vi "CRYSet Auto Save Front Panel.vi"(11 "Vi Ref":refnum<vi>) -> ()   [LabVIEW 2013]
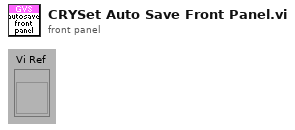
[diagram p1: front panel]
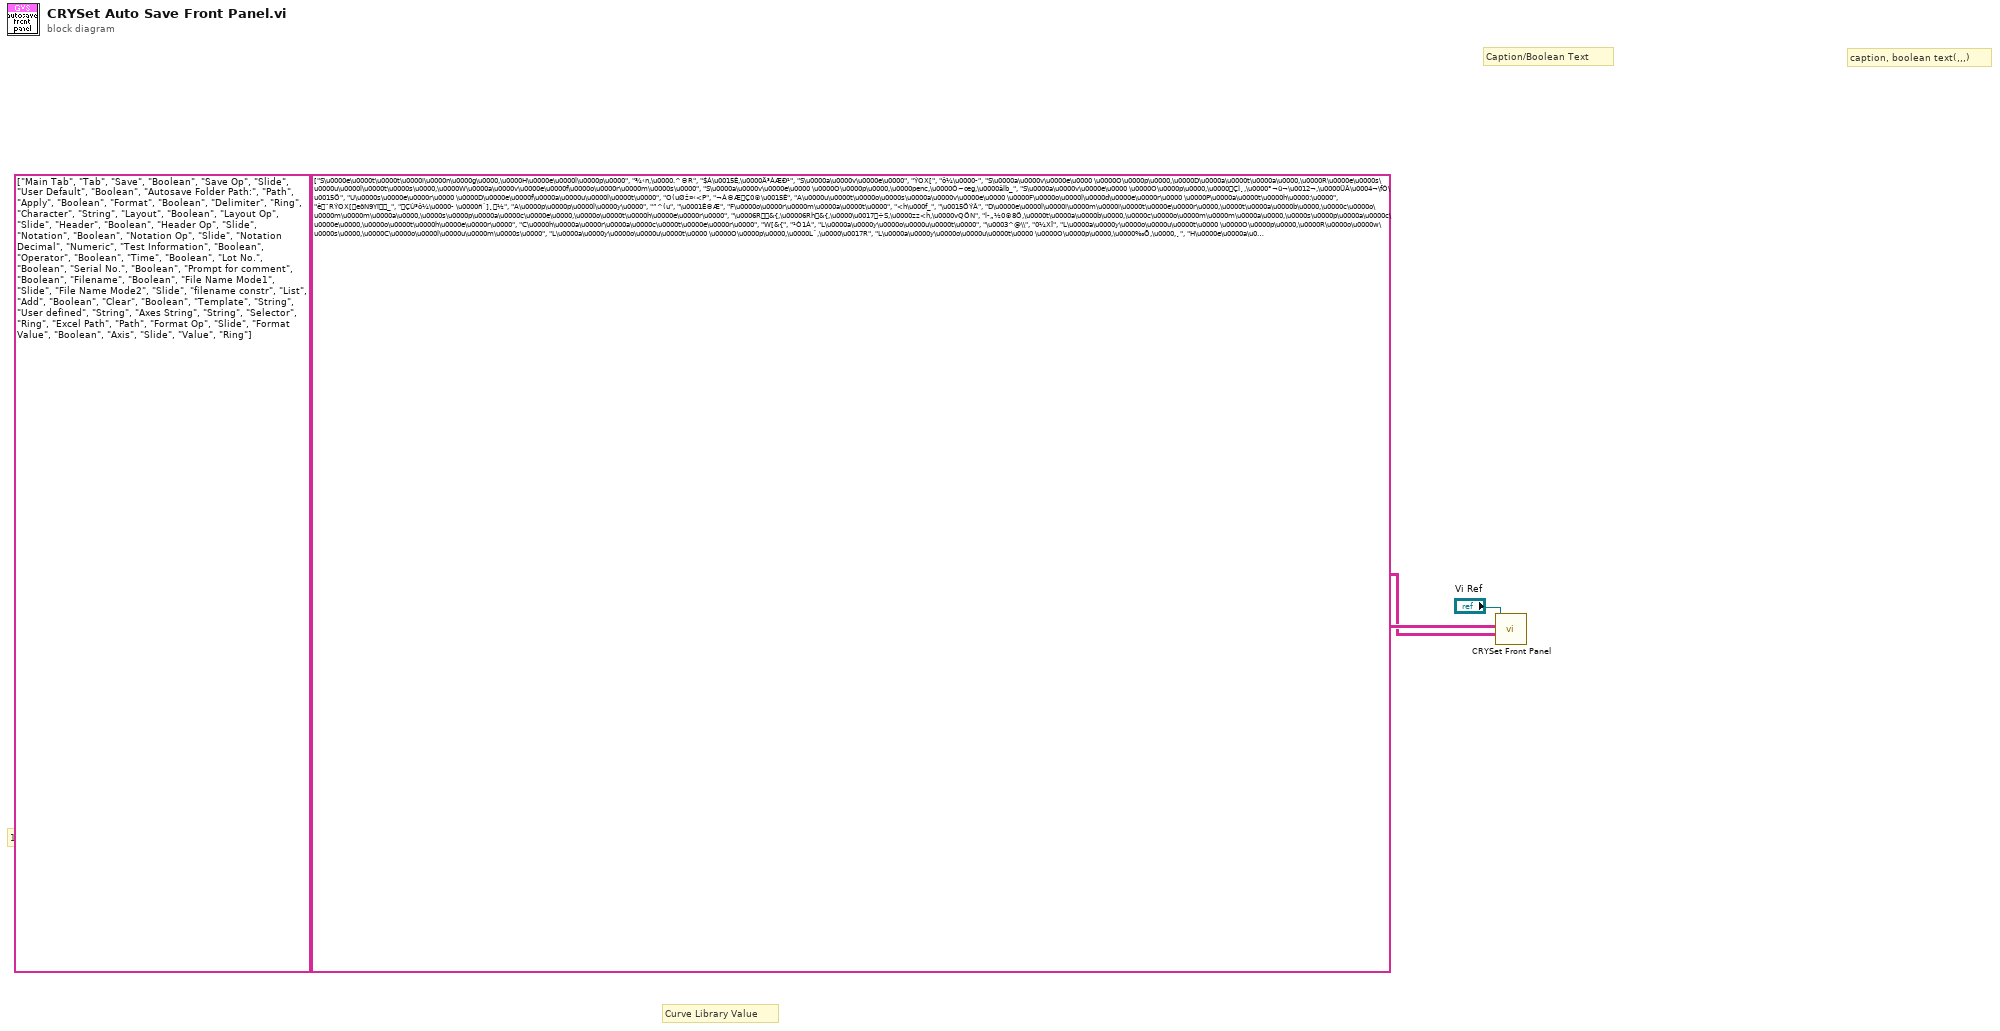
[diagram p0: block diagram]
diagram:
  # "1111"
  # "Curve Library Value"
  # "Caption, Tab Page, Multilist Header, Button 4"
  # "Control Type"
  # "Control Name and Tab"
  # "caption, boolean text(,,,)"
  # "Caption/Boolean Text"
  n1 = call "CRYSet Front Panel.vi"("Caption(Boolean Text)"=string[][] [["S\u0000e\u0000t\u0000t\u0000i\u0000n\u0000g\u0000,\u0000H\u0000e\u0000l\u0000p\u0000", "¾‹n,\u0000.^©R", "$Á\u0015È,\u0000Ä³ÀÆÐ¹"], ["S\u0000a\u0000v\u0000e\u0000", "ÝOX[", "ô¼\u0000­"], ["S\u0000a\u0000v\u0000e\u0000 \u0000O\u0000p\u0000,\u0000D\u0000a\u0000t\u0000a\u0000,\u0000R\u0000e\u0000s\u0000u\u0000l\u0000t\u0000s\u0000,\u0000W\u0000a\u0000v\u0000e\u0000f\u0000o\u0000r\u0000m\u0000s\u0000", "S\u0000a\u0000v\u0000e\u0000 \u0000O\u0000p\u0000,\u0000penc,\u0000Ó~œg,\u0000âlb_", "S\u0000a\u0000v\u0000e\u0000 \u0000O\u0000p\u0000,\u0000ÇÌ¸,\u0000°¬ü¬\u0012¬,\u0000ÜÂ\u0004¬\fÓ\u0015Ö"], ["U\u0000s\u0000e\u0000r\u0000 \u0000D\u0000e\u0000f\u0000a\u0000u\u0000l\u0000t\u0000", "O(uØž¤‹<P", "¬À©ÆÇ0®\u0015È"], ["A\u0000u\u0000t\u0000o\u0000s\u0000a\u0000v\u0000e\u0000 \u0000F\u0000o\u0000l\u0000d\u0000e\u0000r\u0000 \u0000P\u0000a\u0000t\u0000h\u0000:\u0000", "ê¨RÝOX[eöN9Yï_", "ÇÙ³ô¼\u0000­ \u0000ñ´]¸½"], ["A\u0000p\u0000p\u0000l\u0000y\u0000", "”^(u", "\u0001È©Æ"], ["F\u0000o\u0000r\u0000m\u0000a\u0000t\u0000", "<h\u000f_", "\u0015ÖÝÂ"], ["D\u0000e\u0000l\u0000i\u0000m\u0000i\u0000t\u0000e\u0000r\u0000,\u0000t\u0000a\u0000b\u0000,\u0000c\u0000o\u0000m\u0000m\u0000a\u0000,\u0000s\u0000p\u0000a\u0000c\u0000e\u0000,\u0000o\u0000t\u0000h\u0000e\u0000r\u0000", "\u0006R&{,\u00006Rh&{,\u0000\u0017÷S,\u0000zz<h,\u0000vQÖN", "l­„½0®8Ö,\u0000t\u0000a\u0000b\u0000,\u0000c\u0000o\u0000m\u0000m\u0000a\u0000,\u0000s\u0000p\u0000a\u0000c\u0000e\u0000,\u0000o\u0000t\u0000h\u0000e\u0000r\u0000"], ["C\u0000h\u0000a\u0000r\u0000a\u0000c\u0000t\u0000e\u0000r\u0000", "W[&{", "¹Ò1Á"], ["L\u0000a\u0000y\u0000o\u0000u\u0000t\u0000", "\u0003^@\\", "0¼XÎ"], ["L\u0000a\u0000y\u0000o\u0000u\u0000t\u0000 \u0000O\u0000p\u0000,\u0000R\u0000o\u0000w\u0000s\u0000,\u0000C\u0000o\u0000l\u0000u\u0000m\u0000s\u0000", "L\u0000a\u0000y\u0000o\u0000u\u0000t\u0000 \u0000O\u0000p\u0000,\u0000Lˆ,\u0000\u0017R", "L\u0000a\u0000y\u0000o\u0000u\u0000t\u0000 \u0000O\u0000p\u0000,\u0000‰Õ,\u0000,¸"], ["H\u0000e\u0000a\u0000d\u0000e\u0000r\u0000", "\u0007h˜˜", "8º¬¹€½"], ["H\u0000e\u0000a\u0000d\u0000e\u0000r\u0000 \u0000O\u0000p\u0000,\u0000N\u0000o\u0000n\u0000e\u0000,\u0000S\u0000t\u0000a\u0000n\u0000d\u0000a\u0000r\u0000d\u0000,\u0000C\u0000u\u0000s\u0000t\u0000o\u0000m\u0000", "H\u0000e\u0000a\u0000d\u0000e\u0000r\u0000 \u0000O\u0000p\u0000,\u0000àe,\u0000\u0007hÆQ,\u0000ê[IN", "H\u0000e\u0000a\u0000d\u0000e\u0000r\u0000 \u0000O\u0000p\u0000,\u0000ÆÅLÇ,\u0000\\Ô\u0000É,\u0000Ç´Ì\u0015ÈXÇ"], ["N\u0000o\u0000t\u0000a\u0000t\u0000i\u0000o\u0000n\u0000", "&{÷S", "€½8Ö"], ["N\u0000o\u0000t\u0000a\u0000t\u0000i\u0000o\u0000n\u0000 \u0000O\u0000p\u0000,\u0000S\u0000c\u0000i\u0000e\u0000n\u0000t\u0000i\u0000f\u0000i\u0000c\u0000,\u0000F\u0000l\u0000o\u0000a\u0000t\u0000i\u0000n\u0000g\u0000 \u0000p\u0000o\u0000i\u0000n\u0000t\u0000", "N\u0000o\u0000t\u0000a\u0000t\u0000i\u0000o\u0000n\u0000 \u0000O\u0000p\u0000,\u0000Ñyf[,\u0000nm¹p", "N\u0000o\u0000t\u0000a\u0000t\u0000i\u0000o\u0000n\u0000 \u0000O\u0000p\u0000,\u0000ü¬YÕ,\u0000X¹\u0010È"], ["N\u0000o\u0000t\u0000a\u0000t\u0000i\u0000o\u0000n\u0000 \u0000D\u0000e\u0000c\u0000i\u0000m\u0000a\u0000l\u0000", "MO\u000f\\pe", "€½8ÖŒÁ\u0018Â"], ["T\u0000e\u0000s\u0000t\u0000 \u0000I\u0000n\u0000f\u0000o\u0000r\u0000m\u0000a\u0000t\u0000i\u0000o\u0000n\u0000", "KmÕ‹áOo`", "!Î\u0015È\u0015Èô¼"], ["O\u0000p\u0000e\u0000r\u0000a\u0000t\u0000o\u0000r\u0000", "Íd\\OXT", "pÈÇÇ"], ["T\u0000i\u0000m\u0000e\u0000", "öeô•", "ÜÂ\u0004¬"], ["L\u0000o\u0000t\u0000 \u0000N\u0000o\u0000.\u0000", "yb!k", "\u001cÈ‘Çˆ¼8Ö"], ["S\u0000e\u0000r\u0000i\u0000a\u0000l\u0000 \u0000N\u0000o\u0000.\u0000", "^÷S", "Ä¬,¸ˆ¼8Ö"], ["P\u0000r\u0000o\u0000m\u0000p\u0000t\u0000 \u0000f\u0000o\u0000r\u0000 \u0000c\u0000o\u0000m\u0000m\u0000e\u0000n\u0000t\u0000", "èlÊ‘Ðc:y", "üÈtÕ\u001cÈÜÂ"], ["F\u0000i\u0000l\u0000e\u0000n\u0000a\u0000m\u0000e\u0000", "‡eöN\rTðy", "\fÓ|ÇtÇ„¹"], ["F\u0000i\u0000l\u0000e\u0000 \u0000N\u0000a\u0000m\u0000e\u0000 \u0000M\u0000o\u0000d\u0000e\u00001\u0000,\u0000N\u0000e\u0000w\u0000/\u0000O\u0000v\u0000e\u0000r\u0000w\u0000r\u0000i\u0000t\u0000e\u0000,\u0000A\u0000p\u0000p\u0000e\u0000n\u0000d\u0000", "F\u0000i\u0000l\u0000e\u0000 \u0000N\u0000a\u0000m\u0000e\u0000 \u0000M\u0000o\u0000d\u0000e\u00001\u0000,\u0000°e/\u0000†‰Öv,\u0000D– R", "F\u0000i\u0000l\u0000e\u0000 \u0000N\u0000a\u0000m\u0000e\u0000 \u0000M\u0000o\u0000d\u0000e\u00001\u0000,\u0000ÈÀ\\¸/\u0000g³ðÄ0®,\u0000”Í\u0000¬"], ["F\u0000i\u0000l\u0000e\u0000 \u0000N\u0000a\u0000m\u0000e\u0000 \u0000M\u0000o\u0000d\u0000e\u00002\u0000,\u0000A\u0000u\u0000t\u0000o\u0000m\u0000a\u0000t\u0000i\u0000c\u0000,\u0000P\u0000r\u0000o\u0000m\u0000p\u0000t\u0000 \u0000o\u0000p\u0000e\u0000r\u0000a\u0000t\u0000o\u0000r\u0000", "F\u0000i\u0000l\u0000e\u0000 \u0000N\u0000a\u0000m\u0000e\u0000 \u0000M\u0000o\u0000d\u0000e\u00002\u0000,\u0000ê¨R,\u0000Ðc:yÍd\\O", "F\u0000i\u0000l\u0000e\u0000 \u0000N\u0000a\u0000m\u0000e\u0000 \u0000M\u0000o\u0000d\u0000e\u00002\u0000,\u0000ÇÙ³,\u0000pÈÇ\u001cÈÜÂ"], ["C\u0000o\u0000n\u0000s\u0000t\u0000r\u0000u\u0000c\u0000t\u0000i\u0000o\u0000n\u0000", "g ", "l­pÈ"], ["A\u0000d\u0000d\u0000", "ûm R", "¨Ì\u0000¬"], ["C\u0000l\u0000e\u0000a\u0000r\u0000", "\u0005nd–", "­À\u001cÈ"], ["T\u0000e\u0000m\u0000p\u0000l\u0000a\u0000t\u0000e\u0000", "!jg", "\u0015ÖÀÐ"], ["U\u0000s\u0000e\u0000r\u0000 \u0000d\u0000e\u0000f\u0000i\u0000n\u0000e\u0000d\u0000", "(u7bš[IN", "¬À©ÆÇ\u0015ÈXÇ"], ["A\u0000x\u0000e\u0000s\u0000 \u0000S\u0000t\u0000r\u0000i\u0000n\u0000g\u0000,\u0000A\u0000x\u0000e\u0000s\u0000", "A\u0000x\u0000e\u0000s\u0000 \u0000S\u0000t\u0000r\u0000i\u0000n\u0000g\u0000,\u0000t", "A\u0000x\u0000e\u0000s\u0000 \u0000S\u0000t\u0000r\u0000i\u0000n\u0000g\u0000,\u0000•Í"], ["S\u0000e\u0000l\u0000e\u0000c\u0000t\u0000o\u0000r\u0000,\u0000S\u0000p\u0000a\u0000c\u0000e\u0000,\u0000U\u0000n\u0000d\u0000e\u0000r\u0000s\u0000c\u0000o\u0000r\u0000e\u0000s\u0000,\u0000N\u0000o\u0000n\u0000e\u0000", "\téb,\u0000zz<h,\u0000\u000bN\u0012R¿~,\u0000àe", " ÁÝÐÇ,\u0000S\u0000p\u0000a\u0000c\u0000e\u0000,\u0000U\u0000n\u0000d\u0000e\u0000r\u0000s\u0000c\u0000o\u0000r\u0000e\u0000s\u0000,\u0000N\u0000o\u0000n\u0000e\u0000"], ["E\u0000x\u0000c\u0000e\u0000l\u0000 \u0000P\u0000a\u0000t\u0000h\u0000", "h<h!jWeöN9Yï_", "E\u0000x\u0000c\u0000e\u0000l\u0000\u0015ÖÀÐñ´]¸€½"], ["F\u0000o\u0000r\u0000m\u0000a\u0000t\u0000 \u0000O\u0000p\u0000,\u0000T\u0000e\u0000x\u0000t\u0000,\u0000D\u0000A\u0000T\u0000 \u0000R\u0000E\u0000S\u0000 \u0000W\u0000F\u0000M\u0000,\u0000E\u0000x\u0000c\u0000e\u0000l\u0000,\u0000W\u0000A\u0000V\u0000,\u0000D\u0000a\u0000t\u0000a\u0000b\u0000a\u0000s\u0000e\u0000", "F\u0000o\u0000r\u0000m\u0000a\u0000t\u0000 \u0000O\u0000p\u0000,\u0000‡e,g‡eöN,\u0000òf¿~ \u0000Ó~œg \u0000W\u0000F\u0000M\u0000,\u0000E\u0000x\u0000c\u0000e\u0000l\u0000,\u0000W\u0000A\u0000V\u0000,\u0000penc“^", "F\u0000o\u0000r\u0000m\u0000a\u0000t\u0000 \u0000O\u0000p\u0000,\u0000ø¼8»,\u0000\u0012¬ \u0000°¬ü¬ \u0000W\u0000F\u0000M\u0000,\u0000E\u0000x\u0000c\u0000e\u0000l\u0000,\u0000W\u0000A\u0000V\u0000,\u0000ÇÌ¸0®ÀÉ"], ["F\u0000o\u0000r\u0000m\u0000a\u0000t\u0000 \u0000V\u0000a\u0000l\u0000u\u0000e\u0000", "<h\u000f_<P", "\u0015ÖÝÂ\u0012¬"], ["A\u0000x\u0000i\u0000s\u0000,\u0000x\u0000,\u0000y\u0000,\u0000z\u0000", "t,\u0000x\u0000,\u0000y\u0000,\u0000z\u0000", "•Í,\u0000x\u0000,\u0000y\u0000,\u0000z\u0000"], ["C\u0000u\u0000r\u0000v\u0000e\u0000 \u0000L\u0000i\u0000b\u0000r\u0000a\u0000r\u0000y\u0000 \u0000V\u0000a\u0000l\u0000u\u0000e\u0000", "òf¿~“^<P", "á¬ Á\u001cÁà¬\u0012¬"]], "Control ID and Type(Label Name, Type)"=string[][] [["Main Tab", "Tab"], ["Save", "Boolean"], ["Save Op", "Slide"], ["User Default", "Boolean"], ["Autosave Folder Path:", "Path"], ["Apply", "Boolean"], ["Format", "Boolean"], ["Delimiter", "Ring"], ["Character", "String"], ["Layout", "Boolean"], ["Layout Op", "Slide"], ["Header", "Boolean"], ["Header Op", "Slide"], ["Notation", "Boolean"], ["Notation Op", "Slide"], ["Notation Decimal", "Numeric"], ["Test Information", "Boolean"], ["Operator", "Boolean"], ["Time", "Boolean"], ["Lot No.", "Boolean"], ["Serial No.", "Boolean"], ["Prompt for comment", "Boolean"], ["Filename", "Boolean"], ["File Name Mode1", "Slide"], ["File Name Mode2", "Slide"], ["filename constr", "List"], ["Add", "Boolean"], ["Clear", "Boolean"], ["Template", "String"], ["User defined", "String"], ["Axes String", "String"], ["Selector", "Ring"], ["Excel Path", "Path"], ["Format Op", "Slide"], ["Format Value", "Boolean"], ["Axis", "Slide"], ["Value", "Ring"]], "Vi Ref"="Vi Ref") -> ()  [unwired: 9 in]
